vi "FTW-File-Exists.vi"(1 "Filepath":path) -> (0 "Exists?":bool)   [LabVIEW 2012]
panel:
  # "Inputs"
  # "Outputs"
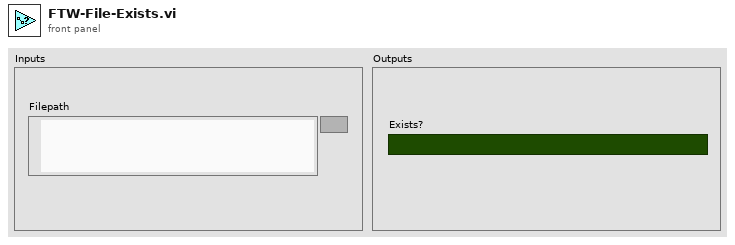
[diagram p1: front panel]
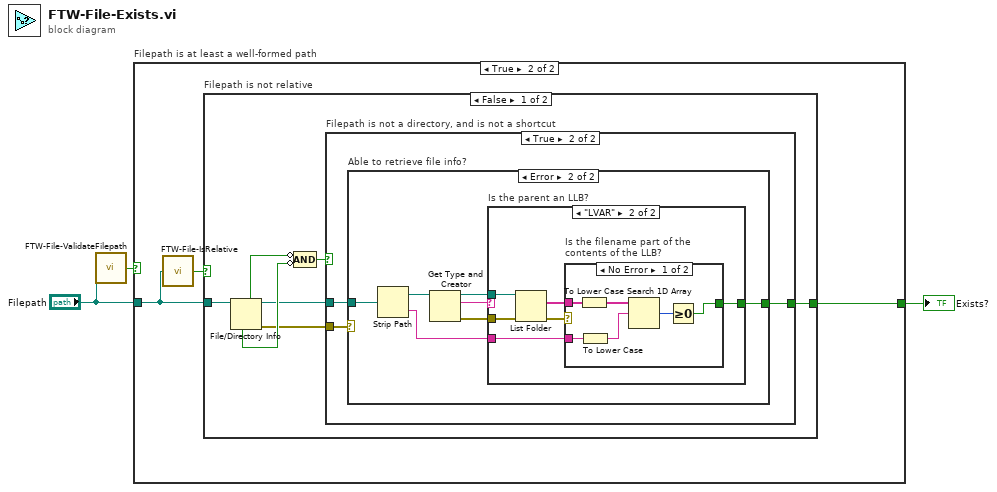
[diagram p0: block diagram]
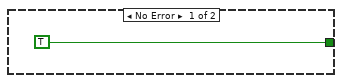
[diagram p4: hidden frame]
diagram:
  n1 = call "FTW-File-ValidateFilepath.vi"("Filepath"="Filepath") -> ("Valid?"=w1:bool)
  n2 = case "Filepath is at least a well-formed path" shown="True" w1 {
    tunnel: "Filepath" -> [_ w5]
    tunnel: [_ w6] -> w3
    frame False {
    }
    frame True {
      n3 = call "FTW-File-IsRelative.vi"("Filepath"=w5) -> ("Relative?"=w4:bool)
      n4 = case "Filepath is not relative" shown="False" w4 {
        tunnel: [w9 _] -> w6
        tunnel: w5 -> [w7 _]
        frame False {
          n5 = File/Directory Info(path=w7) -> (path out=w8:path, directory=w13:bool, error out=w10:errorcluster, shortcut=w12:bool)  [unwired: 1 in, 3 out]
          n6 = Compound Arithmetic op=AND(invert w13, invert w12) -> (w11:bool)
          n7 = case "Filepath is not a directory, and is not a shortcut" shown="True" w11 {
            tunnel: w10 -> [_ w16]
            tunnel: [_ w15] -> w9
            tunnel: w8 -> [_ w14]
            frame False {
            }
            frame True {
              n8 = case "Able to retrieve file info?" shown="Error" w16 {
                tunnel: [TRUE w18] -> w15
                tunnel: w14 -> [_ w21]
                frame No Error {
                }
                frame Error {
                  n9 = Strip Path(path=w21) -> (stripped path=w24:path, name=w23:string)
                  n10 = Get Type and Creator(7:w24) -> (0:w19:errorcluster, 2:w22:string, 3:w20:path)  [unwired: 1 in, 1 out]
                  n11 = case "Is the parent an LLB?" shown="\"LVAR\"" w22 {
                    tunnel: [_ w27] -> w18
                    tunnel: w23 -> [_ w28]
                    tunnel: w20 -> [_ w30]
                    tunnel: w19 -> [_ w26]
                    frame Default {
                    }
                    frame "LVAR" {
                      n12 = List Folder(path=w30, error in=w26) -> (filenames=w29:string[], error out=w25:errorcluster)  [unwired: 4 out]
                      n13 = case "Is the filename part of the\ncontents of the LLB?" shown="No Error" w25 {
                        tunnel: w29 -> [w36 _]
                        tunnel: w28 -> [w35 _]
                        tunnel: [w31 _] -> w27
                        frame No Error {
                          n14 = To Lower Case(string=w36) -> (all lower case string=w33:string[])
                          n15 = To Lower Case(string=w35) -> (all lower case string=w34:string)
                          n16 = Search 1D Array(1D array=w33, element=w34) -> (index of element=w32:i32)  [unwired: 1 out]
                          n17 = Greater Or Equal To 0?(x=w32) -> (x >= 0?=w31:bool)
                        }
                        frame Error {
                        }
                      }
                    }
                  }
                }
              }
            }
          }
        }
        frame True {
        }
      }
    }
  }
  "Exists?" <- w3
